vi "Initialize.vi"(8 "error in (no error)":errorcluster, 11 "Bioreactor in":refnum<class "Bioreactor.lvclass">) -> (0 "error out":errorcluster, 3 "Bioreactor out":refnum<class "Bioreactor.lvclass">)   [LabVIEW 2013, in "Bioreactor.lvlib" / "Bioreactor.lvclass"]
uses:
  Bioreactor.lvclass
  Bioreactor.lvclass/Bioreactor.ctl
  Write Address.vi
  Write VISA resource name.vi
  Read Loop Name.vi
  <vilib>/Instr/_visa.llb/VISA Configure Serial Port (Instr).vi
  PluginInterface/PluginInterface.lvlibp/PluginInterfaceClass/Read TDMS File Path.vi
  PluginInterface/PluginInterface.lvlibp/PluginInterfaceClass/Read DVR.vi
  PluginInterface/PluginInterface.lvlibp/PluginInterfaceClass/Write TDMS.vi
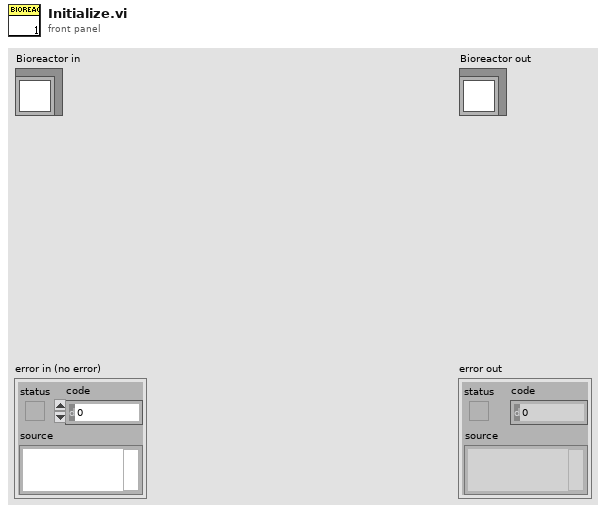
[diagram p1: front panel]
types:
  T1 = enum16{"open", "open or create", "create or replace", "create", "open (read-only)"}
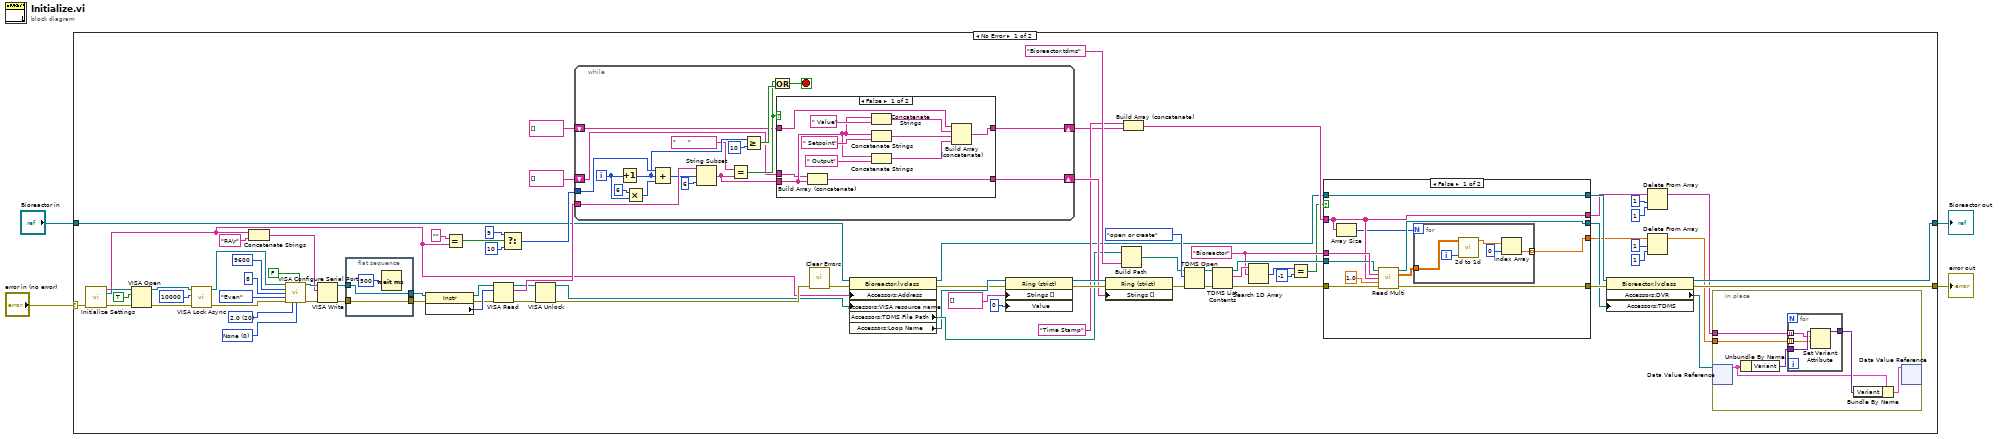
[diagram p0: block diagram]
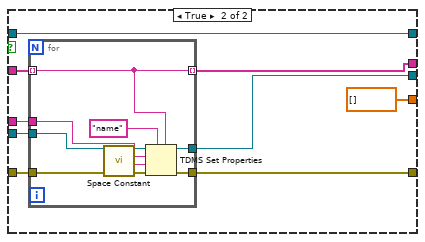
[diagram p2: hidden frame]
diagram:
  n1 = case shown="No Error" "error in (no error)" {
    selector: "error in (no error)" -> [w41 w163]
    tunnel: [w14 w163] -> w3
    tunnel: [w15 w162] -> w1
    tunnel: "Bioreactor in" -> [w39 w162]
    frame No Error {
      w19 = "Bioreactor"
      w75 = u16 0 items=["None", "XON/XOFF", "RTS/CTS", "XON/XOFF & RTS/CTS", "DTR/DSR", "XON/XOFF & DTR/DSR"] ("flow control (0:none)")
      w76 = u16 20 items=["1.0"=10, "1.5"=15, "2.0"=20] ("stop bits (10: 1 bit)")
      n2 = call "Initialize Settings.vi"("error in (no error)"=w41) -> ("Name"=w31:string, "VISA resource name 2"=w47:refnum<visa-resource-name>, "error out"=w48:errorcluster)  [unwired: 12 in]
      n3 = VISA Open(duplicate session (F)=TRUE, error in (no error)=w48, VISA resource name=w47) -> (VISA resource name=w71:refnum<visa-resource-name>, error out=w69:errorcluster)  [unwired: 2 in]
      n4 = call <vilib>:"VISA Lock Async.vi"("error in (no error)"=w69, "timeout (0)"=u32 10000, "VISA resource name"=w71) -> ("error out"=w68:errorcluster, "VISA resource name out"=w70:refnum<visa-resource-name>)  [unwired: 6 in, 1 out]
      n5 = Concatenate Strings(w31, "RA\r") -> (w58:string)
      n6 = call-poly "VISA Configure Serial Port"("VISA resource name"=w70, "Enable Termination\nChar (T)"=FALSE ("Enable Termination Char (T)"), "baud rate (9600)"=9600, "data bits (8)"=8, "parity (0:none)"=enum16{"None", "Odd", "Even", "Mark", "Space"}."Even", "error in (no error)"=w68, "stop bits (10: 1 bit)"=w76, "flow control (0:none)"=w75) -> ("VISA resource name out"=w73:refnum<visa-resource-name>, "error out"=w74:errorcluster)  [unwired: 1 in, 5 out]
      n7 = VISA Write(VISA resource name=w73, write buffer=w58, error in (no error)=w74) -> (VISA resource name out=w63:refnum<visa-resource-name>, error out=w61:errorcluster)  [unwired: 1 out]
      n8 = flat-sequence {
        tunnel: [w161] -> w62
        tunnel: w63 -> [w161]
        tunnel: [w160] -> w60
        tunnel: w61 -> [w160]
        frame #0 {
          n9 = Wait (ms)(milliseconds to wait=500 ("y")) -> ()  [unwired: 1 out]
        }
      }
      n10 = property class="Instr"(reference=w62, error in=w60) -> (reference out=w64:refnum<visa-resource-name>, error out=w65:errorcluster, "Serial Settings:Number of Bytes at Serial Port"=w66:u32)
      n11 = Equal?(x="", y=w31) -> (x = y?=w53:bool)
      n12 = VISA Read(VISA resource name=w64, byte count=w66, error in (no error)=w65) -> (VISA resource name out=w56:refnum<visa-resource-name>, read buffer=w57:string, error out=w55:errorcluster)  [unwired: 1 out]
      n13 = Select(t=9, s=w53, f=10) -> (s? t:f=w49:i32)
      n14 = VISA Unlock(8:w55, 11:w56) -> (0:w42:errorcluster, 3:w32:refnum<visa-resource-name>)
      n15 = while {
        tunnel: w57 -> [w145]
        tunnel: w49 -> [w144]
        shift-right: [w130] -> w29
        shift-left: string[] [] ("appended array") -> [w131]
        shift-right: [w129] -> w45
        shift-left: string[] [] -> [w128]
        i -> [w135]
        stop <- w139 stop-if-true
        n16 = Increment(x=w135) -> (x+1=w142:i32)
        n17 = Multiply(x=6, y=w135) -> (x*y=w134:i32)
        n18 = Compound Arithmetic op=ADD(w144, w142, w134) -> (w143:i32)
        n19 = String Subset(string=w145, offset (0)=w143, length (rest)=6) -> (substring=w137:string)
        n20 = Equal?(x="      " ("y"), y=w137) -> (x = y?=w132:bool)
        n21 = Greater Or Equal?(x=w142, y=10) -> (x >= y?=w140:bool)
        n22 = Or(x=w132, y=w140) -> (x .or. y?=w139:bool)
        n23 = case shown="False" w132 {
          tunnel: w137 -> [w153 _]
          tunnel: w131 -> [w147 w158]
          tunnel: [w146 w158] -> w130
          tunnel: [w151 w157] -> w129
          tunnel: w128 -> [w152 w157]
          frame False {
            n24 = Build Array (concatenate)(w152, w153) -> (w151:string[])
            n25 = Concatenate Strings(w153, " Value" ("string")) -> (w148:string)
            n26 = Concatenate Strings(w153, " Setpoint" ("string")) -> (w149:string)
            n27 = Concatenate Strings(w153, " Output" ("string")) -> (w150:string)
            n28 = Build Array (concatenate)(w147, w148, w149, w150) -> (w146:string[])
          }
          frame True {
          }
        }
      }
      n29 = call <vilib>:"Clear Errors.vi"("error in (no error)"=w42) -> ("error out"=w38:errorcluster)  [unwired: 6 in]
      n30 = property class="Bioreactor.lvclass"(reference=w39, error in=w38, "Accessors:Address"=w31, "Accessors:VISA resource name"=w32) -> (reference out=w17:refnum<class "Bioreactor.lvclass">, error out=w28:errorcluster, "Accessors:TDMS File Path"=w40:path, "Accessors:Loop Name"=w33:refnum<vi>)
      n31 = property class="Ring (strict)"(reference=w33, error in=w28, "Strings []"=string[] [], "Value"=u16 0) -> (reference out=w83:refnum<vi>, error out=w82:errorcluster)
      n32 = property class="Ring (strict)"(reference=w83, error in=w82, "Strings []"=w45) -> (error out=w27:errorcluster)  [unwired: 1 out]
      n33 = Build Path(base path=w40, name or relative path="Bioreactor.tdms") -> (appended path=w44:path)
      n34 = Build Array (concatenate)("Time Stamp" ("Channel"), w29) -> (w18:string[])
      n35 = TDMS Open(8:w27, 10:T1."open or create" ("operation"), 11:w44) -> (0:w23:errorcluster, 3:w22:refnum<k34>)  [unwired: 4 in]
      n36 = TDMS List Contents(4:w23, 7:w22) -> (0:w21:errorcluster, 2:w24:string[], 3:w20:refnum<k34>)  [unwired: 1 in, 1 out]
      n37 = Search 1D Array(1D array=w24, element=w19) -> (index of element=w25:i32)  [unwired: 1 in]
      n38 = Equal?(x=w25, y=-1) -> (x = y?=w13:bool)
      n39 = case shown="False" w13 {
        tunnel: w20 -> [w103 w119]
        tunnel: [w100 w115] -> w36
        tunnel: w21 -> [w104 w117]
        tunnel: w19 -> [w105 w118]
        tunnel: w17 -> [w101 w114]
        tunnel: w18 -> [w97 w116]
        tunnel: [w101 w114] -> w35
        tunnel: [w102 w113] -> w16
        tunnel: [w97 w112] -> w12
        tunnel: [w95 dbl[] []] -> w7
        frame False {
          n40 = Array Size(array=w97) -> (size(s)=w96:i32)
          n41 = call "Read Multi.vi"("tdms file in"=w103, "group"=w105, "Channel"=w97, "Numeric"=1.0, "error in (no error)"=w104) -> ("tdms file out"=w102:refnum<k34>, "Array"=w98:dbl[][], "error out"=w100:errorcluster)  [unwired: 7 in, 1 out]
          n42 = for {
            N: w96 -> [_]
            tunnel: w98 -> [w110]
            tunnel: [w106] -> w95 mode=indexing
            i -> [w107]
            n43 = call "2d to 1d.vi"("index"=w107, "array"=w110) -> ("output array"=w109:dbl[])  [unwired: 9 in]
            n44 = Index Array(array=w109, index=0) -> (element=w106:dbl)
          }
        }
        frame True {
          n45 = for {
            tunnel: w117 -> [w127]
            tunnel: [w126] -> w115
            tunnel: w119 -> [w125]
            tunnel: w118 -> [w124]
            tunnel: w116 -> [w120] mode=indexing
            tunnel: [w121] -> w113
            tunnel: [w120] -> w112 mode=indexing
            n46 = call <vilib>:"Space Constant.vi"() -> ("String"=w122:string)
            n47 = TDMS Set Properties(5:w120, 7:"name" ("property names"), 8:w127, 9:w122, 10:w124, 11:w125) -> (0:w126:errorcluster, 3:w121:refnum<k34>)  [unwired: 2 out]
          }
        }
      }
      n48 = property class="Bioreactor.lvclass"(reference=w35, error in=w36, "Accessors:TDMS"=w16) -> (reference out=w15:refnum<class "Bioreactor.lvclass">, error out=w14:errorcluster, "Accessors:DVR"=w37:refnum<data-value>)
      n49 = Delete From Array(array=w12, length=1, index=1) -> (array with subset deleted=w6:string[])  [unwired: 1 out]
      n50 = Delete From Array(array=w7, length=1, index=1) -> (array with subset deleted=w5:dbl[])  [unwired: 1 out]
      n51 = in-place {
        in-place-border: w6 -> [w86]
        in-place-border: w5 -> [w85]
        n52 = in-place-dvr #1(w37) -> (w87:cluster{"Array":string[], "Variant":variant})  [unwired: 1 out]
        n53 = Unbundle By Name(w87) -> ("Variant"=w89:variant)
        n54 = for {
          tunnel: w89 -> [w94]
          tunnel: [w93] -> w88
          tunnel: w86 -> [w92] mode=indexing
          tunnel: w85 -> [w91] mode=indexing
          n55 = Set Variant Attribute(Variant=w94, name=w92, value=w91) -> (Variant out=w93:variant)  [unwired: 1 in, 2 out]
        }
        n56 = Bundle By Name(cluster=w87, "Variant"=w88) -> (w90:cluster{"Array":string[], "Variant":variant})
        n57 = in-place-dvr #1(w90) -> ()  [unwired: 2 out]
      }
    }
    frame Error {
    }
  }
  "error out" <- w3
  "Bioreactor out" <- w1
